vi "VMSemaphoreAcquire.vi"(8 "error in (no error)":errorcluster, 10 "ms timeout (-1)":i32=-1, 11 "VariableManagerRef in":refnum<vi>) -> (0 "error out":errorcluster, 1 "timed out":bool, 2 "VariableManager":refnum<class "VariableManager.lvclass">, 3 "VariableManagerRef out":refnum<vi>)   [LabVIEW 2013, in "VariableManagerAPI.lvlib"]
doc: "VMSemaphoreAcquire.vi and VMSemaphoreRelease.vi ensure synchronous data operations on a reference to a VariableManager object.\n\nVMSemaphoreAcquire.vi synchronously obtains VariableManager object from the reference for data operations.\nIf other process already acquire semphore of the object, it blocks until the other process call VMSemaphoreRelease.vi or until timed out.\nVMSemaphoreRelease.vi must be called after data operations."
uses:
  VariableManagerAPI.lvlib
  VariableManager/VariableManager.lvclass
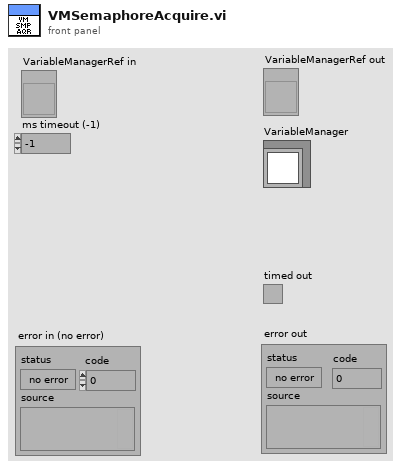
[diagram p1: front panel]
types:
  T1 = typedef "Semaphore RefNum" = refnum<k1>
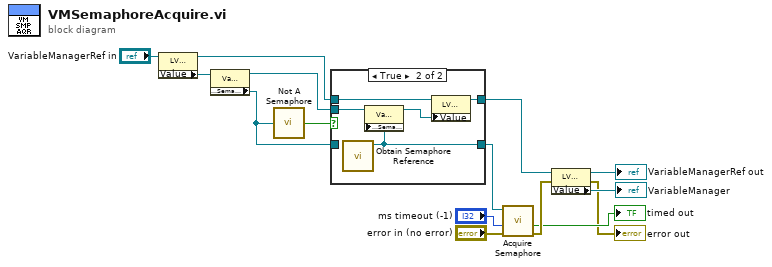
[diagram p0: block diagram]
diagram:
  n1 = property class="LVClassControl (strict)"(reference="VariableManagerRef in") -> (reference out=w15:refnum<vi>, "Value"=w5:refnum<class "VariableManager.lvclass">)  [unwired: 1 in, 1 out]
  n2 = property class="VariableManager.lvclass"(reference=w5) -> (reference out=w14:refnum<class "VariableManager.lvclass">, "Accessors:Semaphore"=w12:T1)  [unwired: 1 in, 1 out]
  n3 = call <vilib>:"Not A Semaphore.vi"("semaphore"=w12) -> ("not a semaphore"=w11:bool)
  n4 = case shown="True" w11 {
    tunnel: w12 -> [w17 _]
    tunnel: [w17 w19] -> w13
    tunnel: w14 -> [_ w22]
    tunnel: w15 -> [w16 w21]
    tunnel: [w16 w18] -> w3
    frame False {
    }
    frame True {
      n5 = call <vilib>:"Obtain Semaphore Reference.vi"() -> ("semaphore"=w19:T1)  [unwired: 5 in, 2 out]
      n6 = property class="VariableManager.lvclass"(reference=w22, "Accessors:Semaphore"=w19) -> (reference out=w20:refnum<class "VariableManager.lvclass">)  [unwired: 1 in, 1 out]
      n7 = property class="LVClassControl (strict)"(reference=w21, "Value"=w20) -> (reference out=w18:refnum<vi>)  [unwired: 1 in, 1 out]
    }
  }
  n8 = call <vilib>:"Acquire Semaphore.vi"("error in (no error)"="error in (no error)", "ms timeout (-1)"="ms timeout (-1)", "semaphore"=w13) -> ("error out"=w9:errorcluster, "timed out"=→"timed out":bool)  [unwired: 2 in, 1 out]
  n9 = property class="LVClassControl (strict)"(reference=w3, error in=w9) -> (reference out=→"VariableManagerRef out":refnum<vi>, error out=→"error out":errorcluster, "Value"=→"VariableManager":refnum<class "VariableManager.lvclass">)
